vi "SVG Parser.vi"(6 "error in (no error)":errorcluster, 9 "XML File Path":path) -> (0 "error out":errorcluster, 1 "paths":T2(array[cluster]), 2 "rects":T3(array[cluster]), 3 "Image Size":cluster{"Width":dbl, "Height":dbl})   [LabVIEW 2011]
doc: "This VI parses an SVG file using LabVIEW's built-in XML parser. It outputs the objects found in an SVG file as well as the canvas width and height."
uses:
  <vilib>/Analysis/Matrix/Datatypes/RealMatrix.ctl
  <vilib>/Analysis/Matrix/NI_Matrix.lvlib
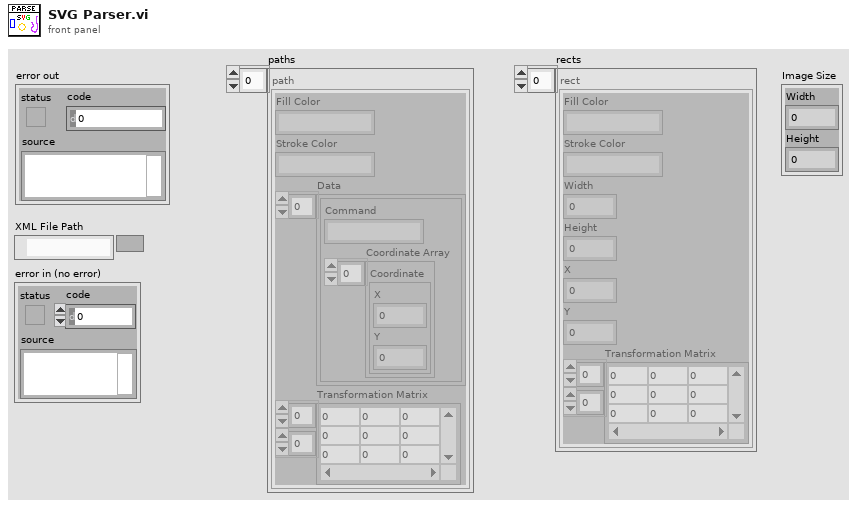
[diagram p1: front panel]
types:
  T1 = typedef "NI_Matrix.lvlib/RealMatrix.ctl" = dbl[][]
  T2 = cluster{"Fill Color":string, "Stroke Color":string, "Data":cluster{"Command":string, "Coordinate Array":cluster{"X":dbl, "Y":dbl}[]}[], "Transformation Matrix":T1}[]
  T3 = cluster{"Fill Color":string, "Stroke Color":string, "Width":dbl, "Height":dbl, "X":dbl, "Y":dbl, "Transformation Matrix":T1}[]
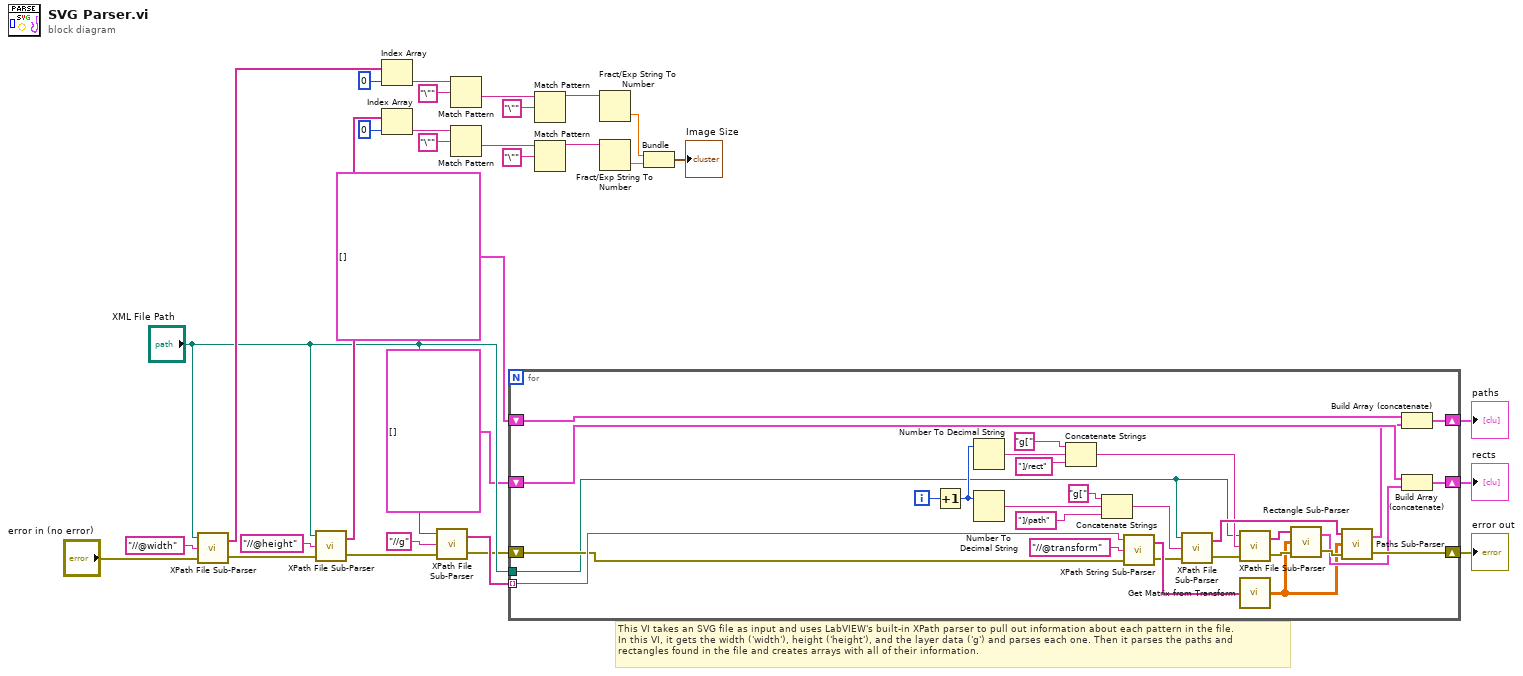
[diagram p0: block diagram]
diagram:
  # "This VI takes an SVG file as input and uses LabVIEW's built-in XPath parser to pull out information about each pattern in the file. \nIn this VI, it gets the width ('width'), height ('height'), and the layer data ('g') and parses each one. Then it parses the paths and \nrectangles found in the file and creates arrays with all of their information."
  n1 = call "XPath File Sub-Parser.vi"("error in (no error)"="error in (no error)", "XPath Expression"="//@width" ("XPath expression"), "XML File Path"="XML File Path") -> ("error out"=w25:errorcluster, "Array of Results"=w30:string[])
  n2 = call "XPath File Sub-Parser.vi"("error in (no error)"=w25, "XPath Expression"="//@height" ("XPath expression"), "XML File Path"="XML File Path") -> ("error out"=w13:errorcluster, "Array of Results"=w27:string[])
  n3 = Index Array(array=w30, index=0) -> (element=w20:string)
  n4 = Index Array(array=w27, index=0) -> (element=w15:string)
  n5 = call "XPath File Sub-Parser.vi"("error in (no error)"=w13, "XPath Expression"="//g" ("XPath expression"), "XML File Path"="XML File Path") -> ("error out"=w10:errorcluster, "Array of Results"=w12:string[])
  n6 = Match Pattern(string=w20, regular expression="\"") -> (after substring=w23:string)  [unwired: 1 in, 3 out]
  n7 = Match Pattern(string=w15, regular expression="\"") -> (after substring=w17:string)  [unwired: 1 in, 3 out]
  n8 = for {
    tunnel: w12 -> [w53] mode=indexing
    tunnel: "XML File Path" -> [w37]
    shift-right: [w54] -> w8
    shift-left: w10 -> [w47]
    shift-right: [w49] -> w7
    shift-left: T3 [] -> [w48]
    shift-right: [w32] -> w6
    shift-left: T2 [] -> [w33]
    i -> [w39]
    n9 = Increment(x=w39) -> (x+1=w38:i32)
    n10 = Number To Decimal String(number=w38) -> (decimal integer string=w41:string)  [unwired: 1 in]
    n11 = Number To Decimal String(number=w38) -> (decimal integer string=w59:string)  [unwired: 1 in]
    n12 = Concatenate Strings("g[" ("string"), w41, "]/rect" ("string")) -> (w40:string)
    n13 = Concatenate Strings("g[" ("string"), w59, "]/path" ("string")) -> (w60:string)
    n14 = call "XPath String Sub-Parser.vi"("error in (no error)"=w47, "XPath expression"="//@transform", "XML String"=w53) -> ("error out"=w46:errorcluster, "Array of Results"=w51:string[])
    n15 = call "XPath File Sub-Parser.vi"("error in (no error)"=w46, "XPath Expression"=w60, "XML File Path"=w37) -> ("error out"=w45:errorcluster, "Array of Results"=w44:string[])
    n16 = call "XPath File Sub-Parser.vi"("error in (no error)"=w45, "XPath Expression"=w40, "XML File Path"=w37) -> ("error out"=w36:errorcluster, "Array of Results"=w55:string[])
    n17 = call "Get Matrix from Transform.vi"("Transform Attributes"=w51) -> ("Matrix"=w35:T1)
    n18 = call "Rectangle Sub-Parser.vi"("error in (no error)"=w36, "Transformation Matrix"=w35, "Array of Nodes"=w55) -> ("error out"=w56:errorcluster, "rects"=w50:T3)
    n19 = call "Paths Sub-Parser.vi"("error in (no error)"=w56, "Transformation Matrix"=w35, "Array of Nodes"=w44) -> ("error out"=w54:errorcluster, "paths"=w34:T2)
    n20 = Build Array (concatenate)(w33, w34) -> (w32:T2)
    n21 = Build Array (concatenate)(w48, w50) -> (w49:T3)
  }
  "error out" <- w8
  "rects" <- w7
  "paths" <- w6
  n22 = Match Pattern(string=w23, regular expression="\"") -> (before substring=w21:string)  [unwired: 1 in, 3 out]
  n23 = Match Pattern(string=w17, regular expression="\"") -> (before substring=w19:string)  [unwired: 1 in, 3 out]
  n24 = Fract/Exp String To Number(string=w21) -> (number=w2:dbl)  [unwired: 3 in, 1 out]
  n25 = Fract/Exp String To Number(string=w19) -> (number=w3:dbl)  [unwired: 3 in, 1 out]
  n26 = Bundle(w2, w3) -> (→"Image Size":cluster{dbl, dbl})  [unwired: 1 in]
